vi "GlobalBaslerCamera.vi"() -> ()   [LabVIEW 2012]
uses:
  <vilib>/userdefined/High Color/IMAQdx.ctl
  <vilib>/vision/Image Controls.llb/IMAQ Image.ctl
panel:
  in  "force background save":bool
  out "image buffering semaphore":T1
  in  "experiment name":string
  in  "number of valid images acquired":i32=5
  out "touching rigth border":bool
  in  "filled buffer":i32=5
  in  "buffer iteration save":i32=5
  in  "buffer index save":i32=5
  in  "buffer iteration":i32=5
  out "rectangle position buffer":u16[][](array[numeric])
  out "image number buffer":u16[](array[numeric])
  in  "buffer index":i32=5
  out "image buffer":T2[](array[typedef])
  in  "buffer size":i32=5
  in  "data path":path
  in  "adjust image":bool
  out "subsampled background":T2
  out "background image":T2
  out "saving background":bool
  in  "BG save time":i64=2500
  in  "sub image height":u32=2500
  in  "sub image width":u32=2500
  in  "temp path":path
  out "error out":errorcluster
  out "Session Out":T3 caption="session"
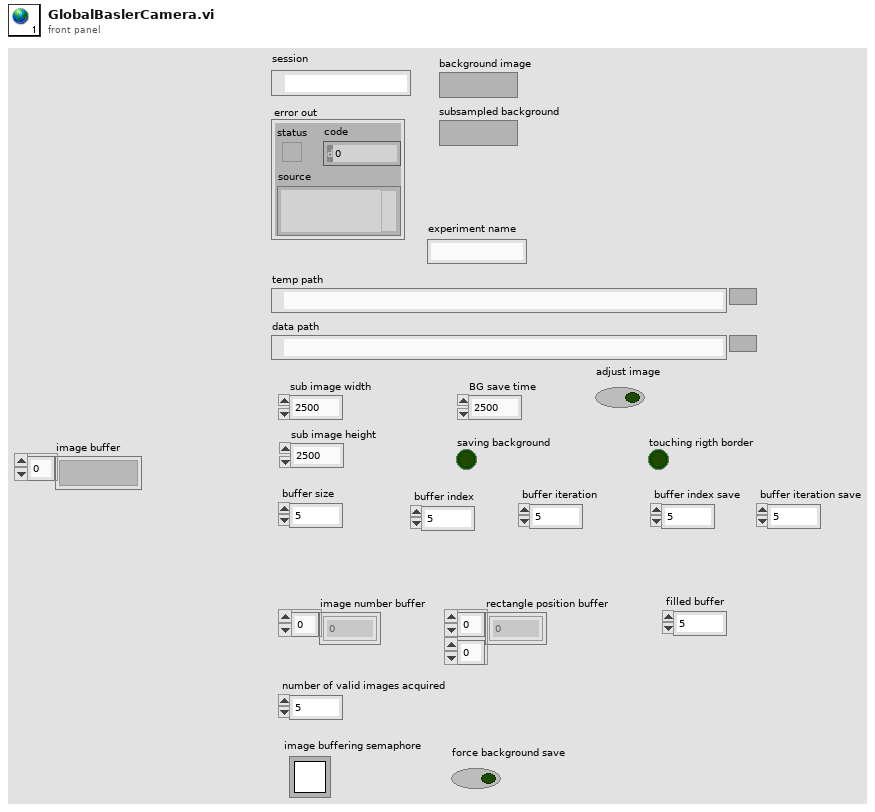
[diagram p1: front panel]
types:
  T1 = typedef "Semaphore RefNum" = refnum<k1>
  T2 = typedef "IMAQ Image.ctl" = refnum<image>
  T3 = typedef "IMAQdx.ctl" = refnum<k21>
diagram:
